vi "SendPacket.vi"(8 "error in":errorcluster, 11 "Packet Array":string[](array[string])) -> (0 "error out":errorcluster, 3 "Time per plane":u32)   [LabVIEW 2017]
uses:
  Typedefs/HW config states enum.ctl
panel:
  out "Ethernet Port Open":bool
  out "FOR Loop":i32
  out "Read Array":string[](array[string])
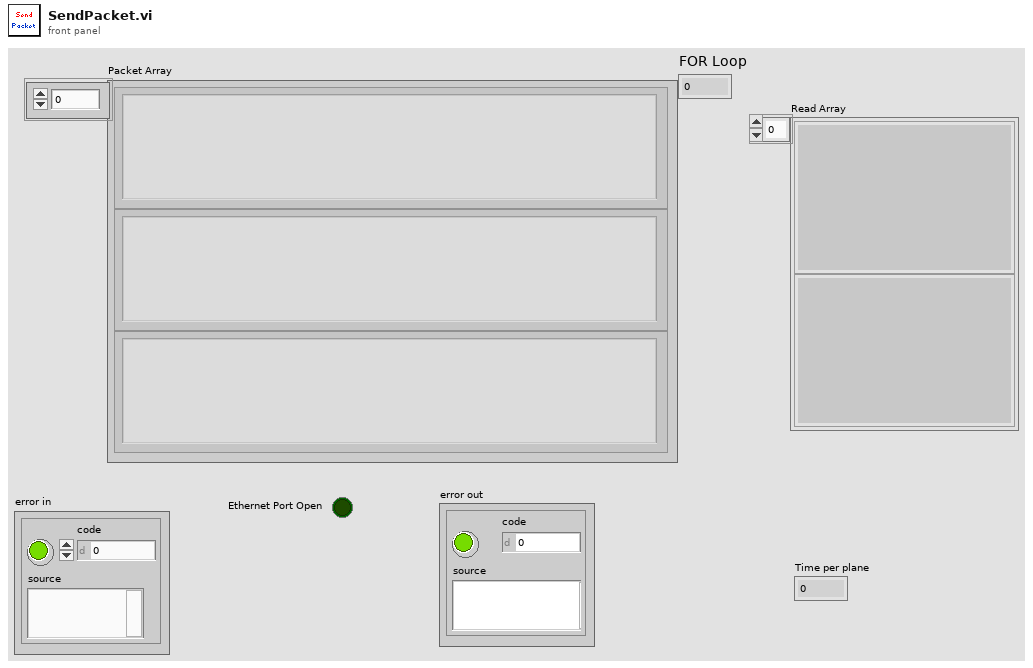
[diagram p1: front panel]
types:
  T1 = typedef "HW config states enum.ctl" = enum16{"Load from file", "Save to file", "Write all", "Read all", "Write XY stage settings", "Write DAQ FPGA settings", "Write Control FPGA settings", "Write Phys Channels", "Clear", "Compare from file"}
  T2 = typedef "Hardware Configuration settings.ctl" = cluster{"Dev. PC":bool, "Swap XY on stage":bool, "No of AOD":u8, "MC Supported":bool, "Axial MC":bool, "Computer MAC address":string, "Externalise Triggers":bool, "Trigger HW config":T3, "DAQmx Chan":T4, "XY stage available":bool, "XY Stage":T5, "Z stage available":bool, "Z Stage config cluster":T6, "Encoder available":bool, "Encoder":T7, "VidRec available":bool, "Cam VidRec":T8, "Laser Power Control HW config":T9, "Laser 1 available":bool, "Laser 1 config cluster":T10, "Prechirper 1 available":bool, "Prechirper 1 config cluster":T11, "Control system.FPGA available?":bool, "Control Sys. HW config":T12, "DAQ FPGA HW Config":T13}
  T3 = typedef "Triggers HW config.ctl" = cluster{"Available Device List":i32, "Device Address":string}
  T4 = typedef "DAQmx physical channels cluster.ctl" = cluster{"Pockels AO":tag, "Hard shutter AO":tag, "PMT AOs":tag, "Galvo AOs":tag, "Power meter AI":tag}
  T5 = typedef "XY Stage config cluster.ctl" = cluster{"COM port":refnum<visa-resource-name>, "XY stage available":bool, "Baudrate":i32, "Type":string}
  T6 = typedef "Z Stage config cluster.ctl" = cluster{"COM port":refnum<visa-resource-name>, "Z stage available":bool, "Baudrate":i32, "Type":string}
  T7 = typedef "Encoder config cluster.ctl" = cluster{"IP address":string, "Port":u16, "Encoder available":bool, "Wheel radius (cm)":dbl, "Encoder Trigger":tag}
  T8 = typedef "Cam VidRec HW config setup cluster.ctl" = cluster{"DO flag-Video record":tag, "DO flag-Trial start":tag, "VidRec available":bool}
  T9 = typedef "Laser Power Control HW config.ctl" = cluster{"Laser Power Control":string, "Laser Power Modulation Control":enum16{"NI", "FPGA"}}
  T10 = typedef "Laser 1 config cluster.ctl" = cluster{"COM port":refnum<visa-resource-name>, "Laser 1 available":bool, "Baud Rate":i32, "Type":string}
  T11 = typedef "PreChirper 1 config cluster.ctl" = cluster{"Type":string, "Baud Rate":i32, "Prechirper 1 available":bool, "COM port":refnum<visa-resource-name>}
  T12 = typedef "Control Sys HW config cluster.ctl" = cluster{"Control system.FPGA available?":bool, "Control system.FPGA Type":enum16{"Virtex 5", "Virtex 7"}, "Control system.Network adapter name":string, "Control system.MAC address":string, "Control system.Ethernet Port":u32, "Control system.Ethernet Port Opened":bool}
  T13 = typedef "DAQ FPGA HW config cluster.ctl" = cluster{"FGPA Ref":T14, "Target":T15, "input card type":T16}
  T14 = typedef "FPGA Ref.ctl" = refnum<k20>
  T15 = typedef "nirio_resource_hc.ctl" = tag
  T16 = typedef "FPGA input type AC-DC.ctl" = enum16{"AC Card", "DC Card"}
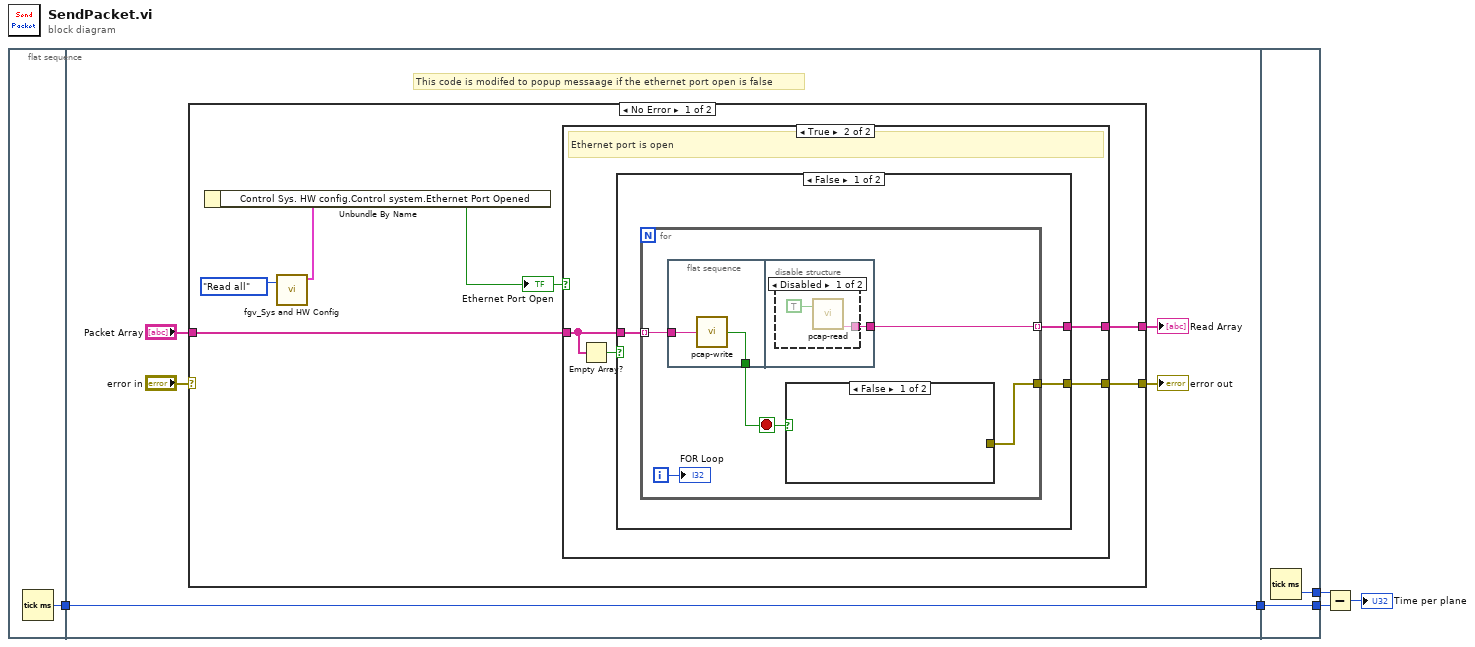
[diagram p0: block diagram]
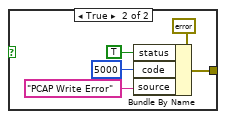
[diagram p3: hidden frame]
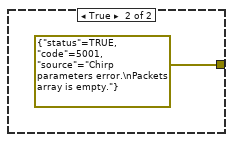
[diagram p5: hidden frame]
diagram:
  n1 = flat-sequence {
    tunnel: [w6] -> w4
    tunnel: w4 -> [w7]
    tunnel: [w7] -> w3
    tunnel: [w43] -> w5
    tunnel: w3 -> [w42]
    tunnel: [w42] -> w2
    frame #0 {
      n2 = Tick Count (ms)() -> (millisecond timer value=w6:u32)
    }
    frame #1 {
      # "This code is modifed to popup messaage if the ethernet port open is false"
      n3 = case shown="No Error" "error in" {
        selector: "error in" -> [_ w41]
        tunnel: "Packet Array" -> [w16 _]
        tunnel: [w17 w41] -> w10
        tunnel: [w15 _] -> w8
        frame No Error {
          n4 = call "fgv_Sys and HW Config.vi"("Function"=HW_config_states_enum."Read all") -> ("Hardware Configuration OUT"=w12:T2)  [unwired: 8 in, 2 out]
          n5 = Unbundle By Name(w12) -> ("Control Sys. HW config.Control system.Ethernet Port Opened"=w13:bool)
          "Ethernet Port Open" <- w13
          n6 = case shown="True" w13 {
            tunnel: [_ w20] -> w17
            tunnel: w16 -> [_ w19]
            tunnel: [_ w21] -> w15
            frame False {
              # "Ethernet port is closed"
            }
            frame True {
              # "Ethernet port is open"
              n7 = Empty Array?(array=w19) -> (empty?=w18:bool)
              n8 = case shown="False" w18 {
                tunnel: w19 -> [w24 _]
                tunnel: [w23 _] -> w21
                tunnel: [w22 errorcluster {"status"=TRUE, "code"=5001, "source"="Chirp parameters error.\nPackets array is empty."} ("error out")] -> w20
                frame False {
                  n9 = for {
                    tunnel: w24 -> [w29] mode=indexing
                    tunnel: [w28] -> w23 mode=indexing
                    tunnel: [w26] -> w22
                    i -> [w27]
                    stop <- w25 stop-if-true
                    n10 = flat-sequence {
                      tunnel: [w36] -> w25
                      tunnel: w29 -> [w35]
                      tunnel: [w37] -> w28
                      frame #0 {
                        n11 = call "pcap-write.vi"("Data to Write"=w35) -> ("Write Error"=w36:bool)
                      }
                      frame #1 {
                        n12 = disable-structure shown="Disabled" {
                          disable-tunnel: [w38 _] -> w37
                          frame Disabled {
                            n13 = call "pcap-read.vi"("Opened"=TRUE) -> ("Packet Data:"=w38:string)  [unwired: 6 out]
                          }
                          frame Enabled {
                          }
                        }
                      }
                    }
                    n14 = case shown="False" w25 {
                      tunnel: [_ w32] -> w26
                      frame False {
                      }
                      frame True {
                        n15 = Bundle By Name(cluster=errorcluster {"status"=FALSE, "code"=0, "source"=""} ("error out"), "status"=TRUE, "code"=5000, "source"="PCAP Write Error") -> (w32:errorcluster)
                      }
                    }
                    "FOR Loop" <- w27
                  }
                }
                frame True {
                }
              }
            }
          }
        }
        frame Error {
        }
      }
      "error out" <- w10
      "Read Array" <- w8
    }
    frame #2 {
      n16 = Tick Count (ms)() -> (millisecond timer value=w43:u32)
    }
  }
  n17 = Subtract(x=w5, y=w2) -> (x-y=→"Time per plane":u32)
